vi "Slave Target.vi"() -> ()   [LabVIEW 2011]
uses:
  Common/controls/Grips Buttons.ctl
  Common/classes/PXI/PXI.lvclass
  Common/controls/Task Definition.ctl
  Common/controls/Task Types.ctl
  Common/classes/GripsMaster/GripsMaster.lvclass
  Common/labview_msgs/sensor_msgs/JointState.ctl
panel:
  in  "ROS IP":string="138.100.76.211"
  out "UDP Status":errorcluster
  in  "ROS Port":u16=5555
  out "Grips Buttons":T1
  in  "Stop":bool
  out "Labview Status":errorcluster
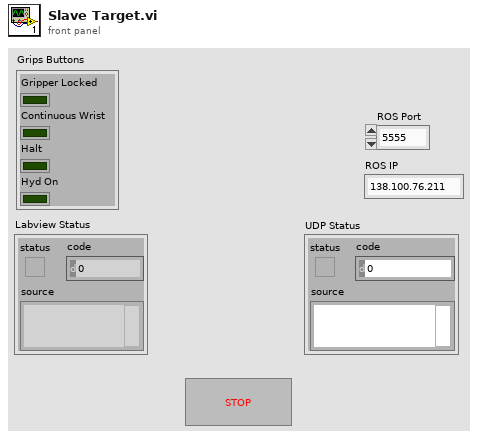
[diagram p1: front panel]
types:
  T1 = typedef "Grips Buttons.ctl" = cluster{"Gripper Locked":bool, "Continuous Wrist":bool, "Halt":bool, "Hyd On":bool}
  T2 = typedef "Task Definition.ctl" = cluster{"task_type":T3, "names":string[], "physical channels":tag, "min_value":dbl, "max_value":dbl, "task_number":i32}
  T3 = typedef "Task Types.ctl" = enum16{"Analog Input", "Analog Output", "Digital Input", "Digital Output"}
  T4 = typedef "Digital Values.ctl" = cluster{"names":string[], "values":bool[]}
  T5 = typedef "Analog Values.ctl" = cluster{"names":string[], "values":dbl[]}
  T6 = enum16{"big-endian, network order", "native, host order", "little-endian"}
  T7 = typedef "JointState.ctl" = cluster{"header":cluster{"seq":u32, "stamp":cluster{"sec":i32, "nsec":i32}, "frame_id":string}, "name":string[], "position":dbl[], "velocity":dbl[], "effort":dbl[]}
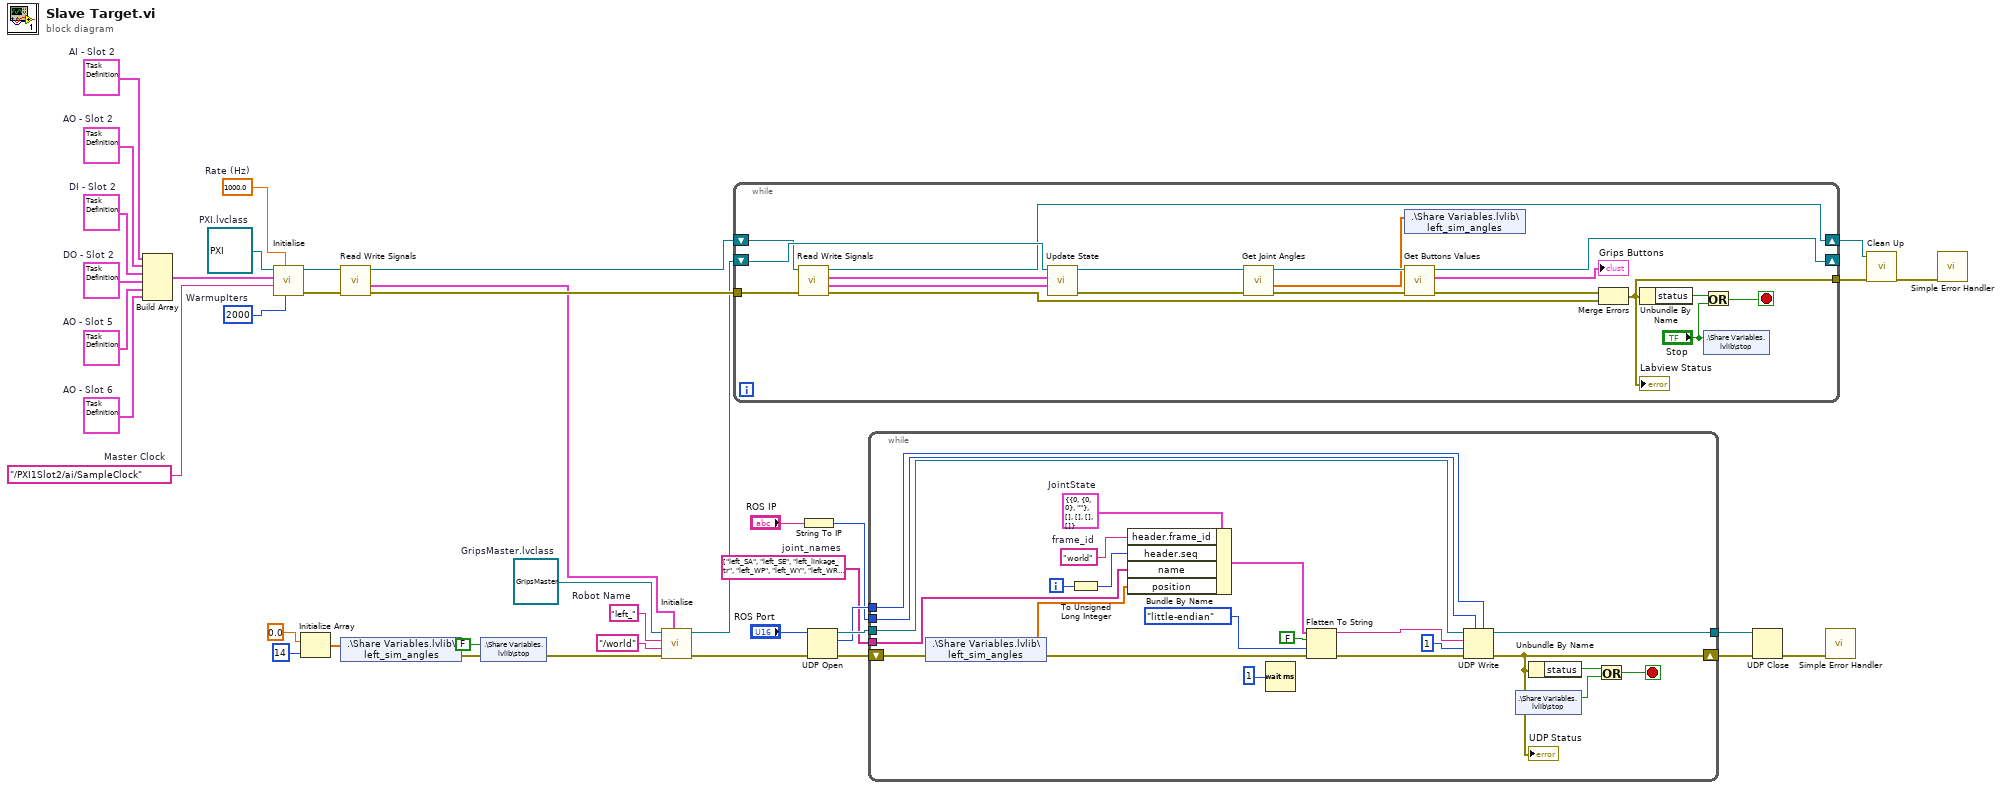
[diagram p0: block diagram]
diagram:
  w10 = string[] ["left_SA", "left_SE", "left_linkage_tr", "left_WP", "left_WY", "left_WR", "left_GRIP", "right_SA", "right_SE", "right_linkage_tr", "right_WP", "right_WY", "right_WR", "right_GRIP"]  # joint_names
  w26 = "left_"  # Robot Name
  w27 = refnum<class "GripsMaster.lvclass"> refnum  # GripsMaster.lvclass
  w39 = 1000.0  # Rate (Hz)
  w30 = u32 2000  # WarmupIters
  w31 = T2 {"task_type"=enum."Analog Output", "names"=["right_WY_FIX", "right_WY_CTR", "right_WP_FIX", "right_WP_CTR", "right_EL_FIX", "right_EL_CTR", "right_SA_FIX", "right_SA_CTR"], "physical channels"="PXI1Slot6/ao0:7", "min_value"=-2.0, "max_value"=2.0, "task_number"=0}  # AO - Slot 6
  w36 = T2 {"task_type"=enum."Analog Output", "names"=["left_WY_FIX", "left_WY_CTR", "left_WP_FIX", "left_WP_CTR", "left_EL_FIX", "left_EL_CTR", "left_SA_FIX", "left_SA_CTR"], "physical channels"="PXI1Slot5/ao0:7", "min_value"=-2.0, "max_value"=2.0, "task_number"=0}  # AO - Slot 5
  w34 = T2 {"task_type"=enum."Analog Output", "names"=["left_SE_FIX", "left_SE_CTR", "right_SE_FIX", "right_SE_CTR"], "physical channels"="PXI1Slot2/ao0:3", "min_value"=-2.0, "max_value"=2.0, "task_number"=0}  # AO - Slot 2
  w32 = T2 {"task_type"=enum."Digital Output", "names"=["left_halt", "left_wrist", "left_hyd", "left_gripper", "right_halt", "right_wrist", "right_hyd", "right_gripper"], "physical channels"="PXI1Slot2/port0/line4:7, PXI1Slot2/port0/line12:15", "min_value"=0.0, "max_value"=0.0, "task_number"=0}  # DO - Slot 2
  w33 = T2 {"task_type"=enum."Digital Input", "names"=["left_gripper", "left_wrist", "left_halt", "left_hyd", "right_gripper", "right_wrist", "right_halt", "right_hyd"], "physical channels"="PXI1Slot2/port0/line0:3, PXI1Slot2/port0/line8:11", "min_value"=0.0, "max_value"=0.0, "task_number"=0}  # DI - Slot 2
  w37 = T2 {"task_type"=enum."Analog Input", "names"=["left_SA", "left_EL", "left_WY", "left_WR", "left_SE", "left_WP", "left_WR_360", "left_GRIP", "right_SA", "right_EL", "right_WY", "right_WR", "right_SE", "right_WP", "right_WR_360", "right_GRIP"], "physical channels"="PXI1Slot2/ai0:3, PXI1Slot2/ai8:11, PXI1Slot2/ai16:19, PXI1Slot2/ai24:27", "min_value"=-10.0, "max_value"=10.0, "task_number"=0}  # AI - Slot 2
  w38 = tag "/PXI1Slot2/ai/SampleClock"  # Master Clock
  w40 = refnum<class "PXI.lvclass"> refnum  # PXI.lvclass
  n1 = Build Array(w37, w34, w33, w32, w36, w31) -> (w35:T2[])
  n2 = call "Initialise.vi"("WarmupIters"=w30, "Rate (Hz)"=w39, "Master Clock"=w38, "Tasks Info"=w35, "PXI in"=w40) -> ("error out"=w28:errorcluster, "PXI out"=w29:refnum<class "PXI.lvclass">)  [unwired: 5 in]
  n3 = Initialize Array(0.0 ("element"), 14 ("dimension size")) -> (w2:dbl[])
  n4 = call "Read Write Signals.vi"("error in (no error)"=w28, "PXI in"=w29) -> ("error out"=w23:errorcluster, "Digital Inputs"=w18:T4, "PXI out"=w24:refnum<class "PXI.lvclass">)  [unwired: 6 in, 1 out]
  n5 = shared-variable ".\\Share Variables.lvlib\\left_sim_angles"(w2) -> (error out=w7:errorcluster)  [unwired: 1 in]
  n6 = shared-variable ".\\Share Variables.lvlib\\stop"(FALSE ("stop"), error in=w7) -> (error out=w5:errorcluster)
  n7 = call "Initialise.vi"("Initial DI"=w18, "error in (no error)"=w5, "Robot Frame"="/world", "Robot Name"=w26, "Master in"=w27) -> ("error out"=w1:errorcluster, "Master out"=w19:refnum<class "GripsMaster.lvclass">)  [unwired: 5 in]
  n8 = while {
    tunnel: w23 -> [w55]
    tunnel: [w48] -> w21
    shift-right: [w54] -> w22
    shift-left: w24 -> [w56]
    shift-right: [w45] -> _
    shift-left: w19 -> [w59]
    stop <- w50 stop-if-true
    n9 = call "Read Write Signals.vi"("error in (no error)"=w55, "PXI in"=w56) -> ("error out"=w53:errorcluster, "Digital Inputs"=w51:T4, "Analog Inputs"=w52:T5, "PXI out"=w54:refnum<class "PXI.lvclass">)  [unwired: 6 in]
    n10 = call "Update State.vi"("Digital Inputs"=w51, "Analog Inputs"=w52, "GripsMaster in"=w59) -> ("error out"=w57:errorcluster, "GripsMaster out"=w58:refnum<class "GripsMaster.lvclass">)  [unwired: 5 in, 2 out]
    n11 = call "Get Joint Angles.vi"("error in (no error)"=w57, "GripsMaster in"=w58) -> ("error out"=w46:errorcluster, "simulator_angles"=w41:dbl[], "GripsMaster out"=w47:refnum<class "GripsMaster.lvclass">)  [unwired: 6 in, 1 out]
    n12 = shared-variable ".\\Share Variables.lvlib\\left_sim_angles"(w41) -> ()  [unwired: 1 in, 1 out]
    n13 = call "Get Buttons Values.vi"("error in (no error)"=w46, "GripsMaster in"=w47) -> ("error out"=w44:errorcluster, "Grips Buttons"=→"Grips Buttons":T1, "GripsMaster out"=w45:refnum<class "GripsMaster.lvclass">)  [unwired: 7 in]
    n14 = Merge Errors(w44, w53) -> (w48:errorcluster)
    "Labview Status" <- w48
    n15 = Unbundle By Name(w48) -> ("status"=w49:bool)
    n16 = Or(x=w49, y="Stop") -> (x .or. y?=w50:bool)
    n17 = shared-variable ".\\Share Variables.lvlib\\stop"("Stop") -> ()  [unwired: 1 in, 1 out]
  }
  n18 = String To IP(1:"ROS IP") -> (0:w8:u32)
  n19 = UDP Open(8:w1, 11:"ROS Port") -> (port=w15:refnum<k16>, 0:w14:errorcluster, 2:w12:u16)  [unwired: 3 out]
  n20 = while {
    tunnel: [w76] -> w16
    tunnel: w15 -> [w75]
    tunnel: w12 -> [w74]
    shift-right: [w73] -> w13
    shift-left: w14 -> [w61]
    tunnel: w10 -> [w66]
    tunnel: w8 -> [w65]
    i -> [w77]
    stop <- w71 stop-if-true
    w64 = T7 {"header"={"seq"=0, "stamp"={"sec"=0, "nsec"=0}, "frame_id"=""}, "name"=[], "position"=[], "velocity"=[], "effort"=[]}  # JointState
    w68 = "world"  # frame_id
    n21 = shared-variable ".\\Share Variables.lvlib\\left_sim_angles"(error in=w61) -> (w62:dbl[], error out=w60:errorcluster)
    n22 = To Unsigned Long Integer(number=w77) -> (unsigned 32bit integer=w69:u32)
    n23 = Bundle By Name(cluster=w64, "header.frame_id"=w68, "header.seq"=w69, "name"=w66, "position"=w62) -> (w78:T7)
    n24 = Wait (ms)(milliseconds to wait=u32 1) -> ()  [unwired: 1 out]
    n25 = Flatten To String(anything=w78, prepend array or string size? (T)=FALSE, byte order (0:big-endian, network order)=T6."little-endian" ("Byte order"), error in (no error)=w60) -> (data string=w81:string, error out=w79:errorcluster)  [unwired: 1 out]
    n26 = UDP Write(address=w65, port or service name=w74, connection ID=w75, data in=w81, 8:w79, 9:1 ("timeout ms (25000)")) -> (error out=w73:errorcluster, 3:w76:refnum<k16>)
    "UDP Status" <- w73
    n27 = shared-variable ".\\Share Variables.lvlib\\stop"() -> (w63:bool)  [unwired: 1 in, 1 out]
    n28 = Unbundle By Name(w73) -> ("status"=w72:bool)
    n29 = Or(x=w72, y=w63) -> (x .or. y?=w71:bool)
  }
  n30 = UDP Close(connection ID=w16, 8:w13) -> (error out=w11:errorcluster)  [unwired: 1 out]
  n31 = call <vilib>:"Simple Error Handler.vi"("error in (no error)"=w11) -> ()  [unwired: 4 in, 5 out]
  n32 = call "Clean Up.vi"("error in (no error)"=w21, "PXI in"=w22) -> ("error out"=w20:errorcluster)  [unwired: 8 in, 1 out]
  n33 = call <vilib>:"Simple Error Handler.vi"("error in (no error)"=w20) -> ()  [unwired: 4 in, 5 out]
